vi "Untitled 1.vi"() -> ()   [LabVIEW 2014]
panel:
  out "x*y":i32[][](array[numeric])
  in  "column":i32
  in  "row":i32
  # "Siavash Aghajani"
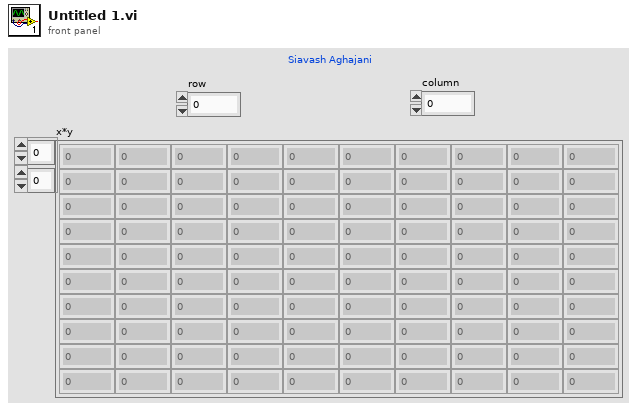
[diagram p1: front panel]
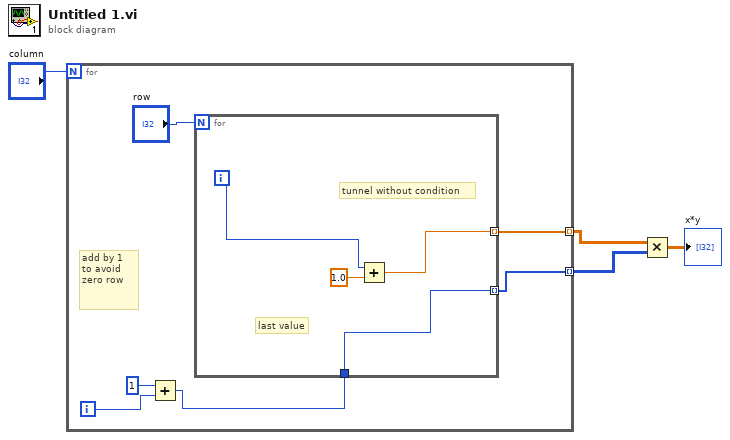
[diagram p0: block diagram]
diagram:
  n1 = for {
    N: "column" -> [_]
    tunnel: [w9] -> w3 mode=indexing
    tunnel: [w5] -> w1 mode=indexing
    i -> [w8]
    # "add by 1  to avoid zero row"
    n2 = Add(x=1, y=w8) -> (x+y=w6:i32)
    n3 = for {
      N: "row" -> [_]
      tunnel: [w12] -> w9 mode=indexing
      tunnel: w6 -> [w12]
      tunnel: [w11] -> w5 mode=indexing
      i -> [w13]
      # "tunnel without condition"
      # "last value"
      n4 = Add(x=w13, y=1.0) -> (x+y=w11:dbl)
    }
  }
  n5 = Multiply(x=w1, y=w3) -> (x*y=→"x*y":dbl[][])
